vi "gfitsio-check-col-for-write.vi"(4 "units":string, 5 "cfitsio datatype":T1=82 items=["TBIT"=1, "TBYTE  (U8)"=11, "TSBYTE  (I8)"=12, "TLOGICAL"=14, "TSTRING"=16, "TUSHORT  (U16)"=20, "TSHORT  (I16)"=21, "TUINT"=31, "TULONG  (U32)"=40, "TLONG  (I32)"=41, "TFLOAT  (SGL)"=42, "TLONGLONG  (I64)"=81, "TDOUBLE  (DBL)"=82, "TCOMPLEX  (CSG)"=83, "TDOUBLECOMPLEX  (CDB)"=163], 6 "row":i32, 7 "column":string, 8 "error in (no error)":errorcluster, 9 "size (-1:variable)":i32=-1, 11 "gfits refnum":T2=refnum) -> (0 "error out":errorcluster, 2 "colnum":i32, 3 "dup gfits refnum":T2)   [LabVIEW 2019, in "gfitsio.lvlib"]
uses:
  gfitsio.lvlib
  gfitsio-refnum.ctl
  cfitsio-datatypes.ctl
  cfitsio-hdutypes.ctl
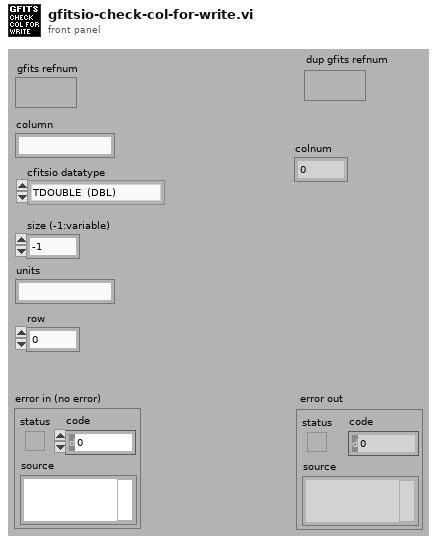
[diagram p1: front panel]
types:
  T1 = typedef "gfitsio.lvlib/cfitsio-datatypes.ctl" = i32
  T2 = typedef "gfitsio.lvlib/gfitsio-refnum.ctl" = refnum<k1>
  T3 = typedef "gfitsio.lvlib/cfitsio-hdutypes.ctl" = i32
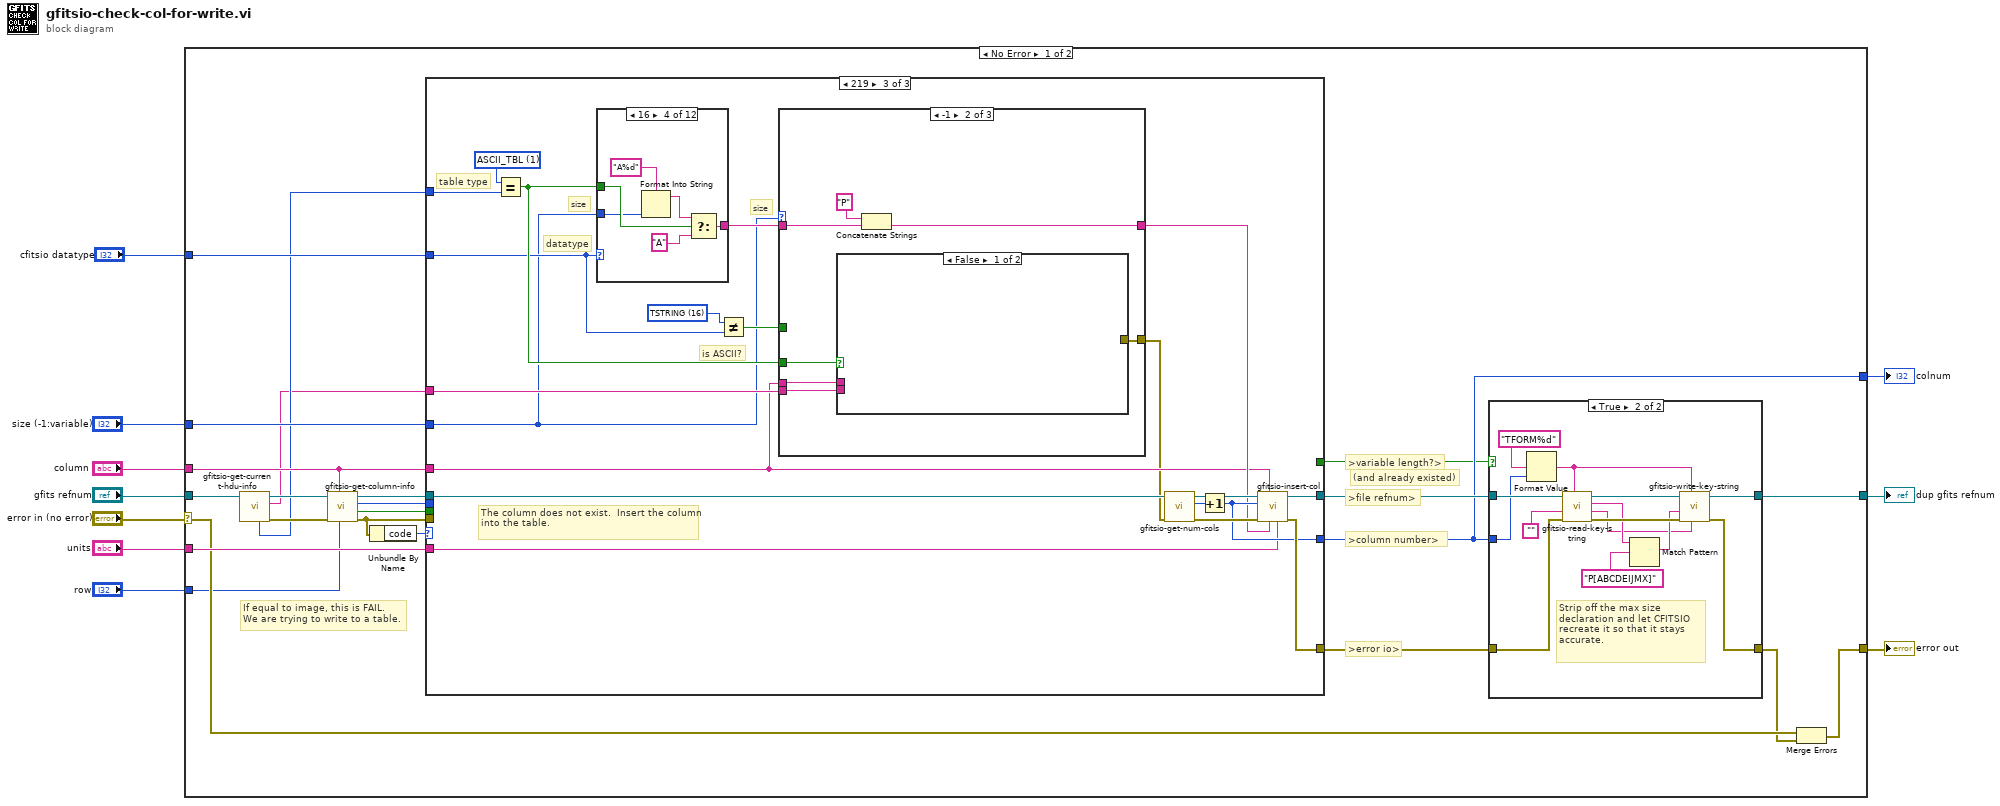
[diagram p0: block diagram]
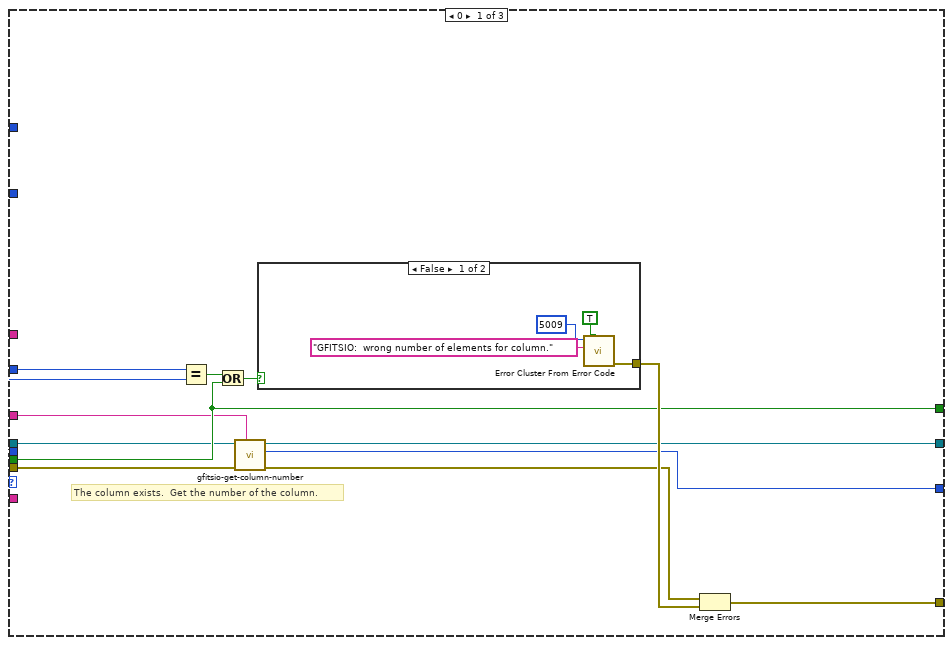
[diagram p2: hidden frame]
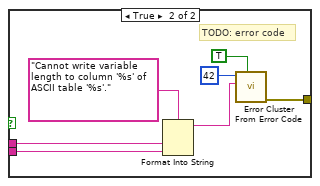
[diagram p6: hidden frame]
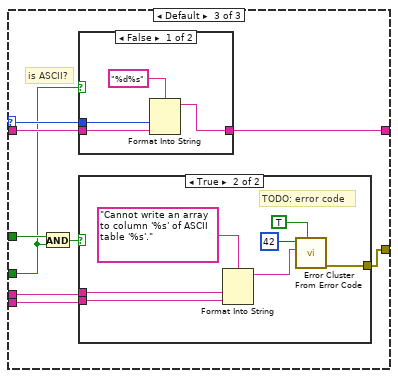
[diagram p7: hidden frame]
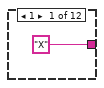
[diagram p10: hidden frame]
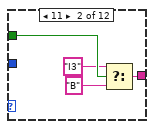
[diagram p11: hidden frame]
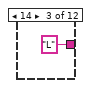
[diagram p12: hidden frame]
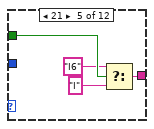
[diagram p13: hidden frame]
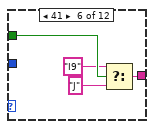
[diagram p14: hidden frame]
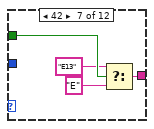
[diagram p15: hidden frame]
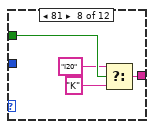
[diagram p16: hidden frame]
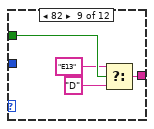
[diagram p17: hidden frame]
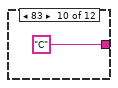
[diagram p18: hidden frame]
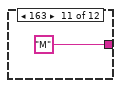
[diagram p19: hidden frame]
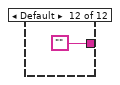
[diagram p20: hidden frame]
diagram:
  n1 = case shown="No Error" "error in (no error)" {
    selector: "error in (no error)" -> [w17 w162]
    tunnel: "units" -> [w33 _]
    tunnel: "column" -> [w32 _]
    tunnel: "size (-1:variable)" -> [w31 _]
    tunnel: "cfitsio datatype" -> [w30 _]
    tunnel: [w16 w162] -> w6
    tunnel: [w27 w161] -> w5
    tunnel: [w26 0 ("colnum")] -> w4
    tunnel: "gfits refnum" -> [w20 w161]
    tunnel: "row" -> [w12 _]
    frame No Error {
      # "(and already existed)"
      # "If equal to image, this is FAIL.\nWe are trying to write to a table."
      # ">error io>"
      # ">file refnum>"
      # ">column number>"
      # ">variable length?>"
      n2 = call "gfitsio-get-current-hdu-info.vi"("gfits refnum"=w20) -> ("error out"=w18:errorcluster, "hdu name"=w13:string, "dup gfits refnum"=w19:T2, "hdu type"=w14:T3)  [unwired: 1 in, 6 out]
      n3 = call "gfitsio-get-column-info.vi"("row (-1: don't check descriptor)"=w12, "column"=w32, "error in (no error)"=w18, "gfits refnum"=w19) -> ("error out"=w23:errorcluster, "variable length array?"=w11:bool, "nelements"=w21:i32, "dup gfits refnum"=w22:T2)  [unwired: 2 in, 2 out]
      n4 = Unbundle By Name(w23) -> ("code"=w24:i32)
      n5 = case shown="219" w24 {
        tunnel: w23 -> [w39 w52 _]
        tunnel: [w42 w52 w72] -> w29
        tunnel: [w36 w51 w71] -> w28
        tunnel: w22 -> [w38 w51 w68]
        tunnel: [w34 _ w66] -> w26
        tunnel: w33 -> [_ _ w63]
        tunnel: w21 -> [w41 _ _]
        tunnel: w31 -> [w46 _ w53]
        tunnel: w30 -> [_ _ w56]
        tunnel: [w40 _ _] -> w25
        tunnel: w32 -> [w37 _ w58]
        tunnel: w11 -> [w40 _ _]
        tunnel: w14 -> [_ _ w62]
        tunnel: w13 -> [_ _ w59]
        frame 0 {
          # "The column exists.  Get the number of the column."
          n6 = Equal?(x=w46, y=w41) -> (x = y?=w45:bool)
          n7 = Or(x=w45, y=w40) -> (x .or. y?=w44:bool)
          n8 = call "gfitsio-get-column-number.vi"("column"=w37, "error in (no error)"=w39, "gfits refnum"=w38) -> ("error out"=w35:errorcluster, "colnum"=w34:i32, "dup gfits refnum"=w36:T2)  [unwired: 1 in, 5 out]
          n9 = case shown="False" w44 {
            tunnel: [w48 _] -> w43
            frame False {
              n10 = call <vilib>:"Error Cluster From Error Code.vi"("show call chain? (False)"=TRUE, "error message (\"\")"="GFITSIO:  wrong number of elements for column." ("error message (\"\")"), "error code (0)"=5009) -> ("error out"=w48:errorcluster)  [unwired: 1 in, 5 out]
            }
            frame True {
            }
          }
          n11 = Merge Errors(w35, w43) -> (w42:errorcluster)
        }
        frame Default {
          # "An error already exists.  Do nothing."
        }
        frame 219 {
          w55 = T1 16 items=["TBIT"=1, "TBYTE  (U8)"=11, "TSBYTE  (I8)"=12, "TLOGICAL"=14, "TSTRING"=16, "TUSHORT  (U16)"=20, "TSHORT  (I16)"=21, "TUINT"=31, "TULONG  (U32)"=40, "TLONG  (I32)"=41, "TFLOAT  (SGL)"=42, "TLONGLONG  (I64)"=81, "TDOUBLE  (DBL)"=82, "TCOMPLEX  (CSG)"=83, "TDOUBLECOMPLEX  (CDB)"=163] ("x")
          w61 = T3 1 items=["ANY_HDU"=-1, "IMAGE_HDU"=0, "ASCII_TBL"=1, "BINARY_TBL"=2] ("x")
          # "is ASCII?"
          # "datatype"
          # "size"
          # "table type"
          # "size"
          # "The column does not exist.  Insert the column into the table."
          n12 = Equal?(x=w61, y=w62) -> (x = y?=w60:bool)
          n13 = case shown="16" w56 {
            tunnel: ["X" ("t") w110 "L" ("t") w119 w121 w125 w129 w133 w137 "C" ("t") "M" ("t") ""] -> w65
            tunnel: w60 -> [_ w113 _ w116 w124 w128 w132 w136 w140 _ _ _]
            tunnel: w53 -> [_ _ _ w115 _ _ _ _ _ _ _ _]
            frame 1 {
            }
            frame 11 {
              n14 = Select(t="I3", s=w113, f="B") -> (s? t:f=w110:string)
            }
            frame 14 {
            }
            frame 16 {
              n15 = Format Into String(format string="A%d", w115) -> (resulting string=w117:string)  [unwired: 2 in, 1 out]
              n16 = Select(t=w117, s=w116, f="A") -> (s? t:f=w119:string)
            }
            frame 21 {
              n17 = Select(t="I6", s=w124, f="I") -> (s? t:f=w121:string)
            }
            frame 41 {
              n18 = Select(t="I9", s=w128, f="J") -> (s? t:f=w125:string)
            }
            frame 42 {
              n19 = Select(t="E13", s=w132, f="E") -> (s? t:f=w129:string)
            }
            frame 81 {
              n20 = Select(t="I20", s=w136, f="K") -> (s? t:f=w133:string)
            }
            frame 82 {
              n21 = Select(t="E13", s=w140, f="D") -> (s? t:f=w137:string)
            }
            frame 83 {
            }
            frame 163 {
            }
            frame Default {
            }
          }
          n22 = Not Equal?(x=w55, y=w56) -> (x != y?=w54:bool)
          n23 = case shown="-1" w53 {
            selector: w53 -> [_ _ w92]
            tunnel: w65 -> [w73 w80 w94]
            tunnel: [w73 w78 w93] -> w64
            tunnel: w60 -> [_ w77 w88]
            tunnel: w59 -> [_ w74 w89]
            tunnel: w58 -> [_ w75 w96]
            tunnel: [_ w76 w95] -> w57
            tunnel: w54 -> [_ _ w91]
            frame 1 {
            }
            frame -1 {
              n24 = case shown="False" w77 {
                tunnel: w75 -> [_ w87]
                tunnel: w74 -> [_ w86]
                tunnel: [_ w81] -> w76
                frame False {
                }
                frame True {
                  # "TODO: error code"
                  n25 = Format Into String(format string="Cannot write variable length to column '%s' of ASCII table '%s'.", w87, w86) -> (resulting string=w83:string)  [unwired: 2 in, 1 out]
                  n26 = call <vilib>:"Error Cluster From Error Code.vi"("show call chain? (False)"=TRUE, "error message (\"\")"=w83, "error code (0)"=42) -> ("error out"=w81:errorcluster)  [unwired: 6 in]
                }
              }
              n27 = Concatenate Strings("P" ("string"), w80) -> (w78:string)
            }
            frame Default {
              # "is ASCII?"
              n28 = And(x=w91, y=w88) -> (x .and. y?=w90:bool)
              n29 = case shown="False" w88 {
                tunnel: w94 -> [w99 w101]
                tunnel: [w98 w101] -> w93
                tunnel: w92 -> [w97 _]
                frame False {
                  n30 = Format Into String(format string="%d%s" ("initial string"), w97, w99) -> (resulting string=w98:string)  [unwired: 2 in, 1 out]
                }
                frame True {
                }
              }
              n31 = case shown="True" w90 {
                tunnel: w96 -> [_ w103]
                tunnel: [_ w104] -> w95
                tunnel: w89 -> [_ w102]
                frame False {
                }
                frame True {
                  # "TODO: error code"
                  n32 = Format Into String(format string="Cannot write an array to column '%s' of ASCII table '%s'.", w103, w102) -> (resulting string=w106:string)  [unwired: 2 in, 1 out]
                  n33 = call <vilib>:"Error Cluster From Error Code.vi"("show call chain? (False)"=TRUE, "error message (\"\")"=w106, "error code (0)"=42) -> ("error out"=w104:errorcluster)  [unwired: 6 in]
                }
              }
            }
          }
          n34 = call "gfitsio-get-num-cols.vi"("error in (no error)"=w57, "gfits refnum"=w68) -> ("error out"=w70:errorcluster, "number of columns"=w69:i32, "dup gfits refnum"=w67:T2)  [unwired: 7 out]
          n35 = Increment(x=w69) -> (x+1=w66:i32)
          n36 = call "gfitsio-insert-col.vi"("tunits"=w63, "tform"=w64, "ttype"=w58, "error in (no error)"=w70, "insertion point (0:1st column)"=w66, "gfits refnum"=w67) -> ("error out"=w72:errorcluster, "dup gfits refnum"=w71:T2)  [unwired: 4 out]
        }
      }
      n37 = case shown="True" w25 {
        tunnel: [w144 w159] -> w15
        tunnel: w29 -> [w144 w156]
        tunnel: w28 -> [w145 w155]
        tunnel: [w145 w154] -> w27
        tunnel: w26 -> [_ w150]
        frame False {
        }
        frame True {
          # "Strip off the max size declaration and let CFITSIO recreate it so that it stays accurate."
          n38 = Format Value(format string="TFORM%d", value (0)=w150) -> (output string=w147:string)  [unwired: 1 out]
          n39 = call "gfitsio-read-key-string.vi"("keyname"=w147, "error in (no error)"=w156, "default value"="", "gfits refnum"=w155) -> ("error out"=w157:errorcluster, "comment"=w146:string, "value"=w149:string, "dup gfits refnum"=w158:T2)  [unwired: 4 out]
          n40 = Match Pattern(string=w149, regular expression="P[ABCDEIJMX]") -> (match substring=w148:string)  [unwired: 4 out]
          n41 = call "gfitsio-write-key-string.vi"("comment"=w146, "keyname"=w147, "error in (no error)"=w157, "value"=w148, "gfits refnum"=w158) -> ("error out"=w159:errorcluster, "dup gfits refnum"=w154:T2)  [unwired: 1 in, 4 out]
        }
      }
      n42 = Merge Errors(w17, w15) -> (w16:errorcluster)
    }
    frame Error {
    }
  }
  "error out" <- w6
  "dup gfits refnum" <- w5
  "colnum" <- w4
